vi "stopInPreparePass.vi"(4 "Game in":refnum<class "Game.lvclass">, 7 "OffensivePlay":T1=enum."TestPlay", 8 "error in (no error)":errorcluster, 9 "Ball":refnum<class "Ball.lvclass">, 10 "Robot in":refnum<class "Robot.lvclass">, 11 "AttackerStopTactic in":refnum<class "AttackerStopTactic.lvclass">) -> (0 "error out":errorcluster, 2 "Robot out":refnum<class "Robot.lvclass">, 3 "AttackerStopTactic out":refnum<class "AttackerStopTactic.lvclass">)   [LabVIEW 2023, in "AttackerStopTactic.lvclass"]
uses:
  AttackerStopTactic.lvclass
  Robot_class/Robot.lvclass
  C:/Users/ebert/Desktop/roboime/SSL_AI/Object_class/Object.lvclass
  Ball_class/Ball.lvclass
  Team_class/OffensivePlay.ctl
  Game_class/Game.lvclass
  Utilities_class/Utilities.lvclass
  Game_class/Game.lvclass/Game.ctl
  Object_class/Object.lvclass/Object.ctl
  Robot_class/Robot.lvclass/Robot.ctl
  <vilib>/Analysis/baseanly.llb/Unit Vector (DBL).vi
  Object_class/Read position(x,y).vi
  Object_class/Read y.vi
  Robot_class/Write dest_x.vi
  Robot_class/Write dest_y.vi
  Game_class/Read NewParameters.vi
  <vilib>/Analysis/NI_AALBase.lvlib
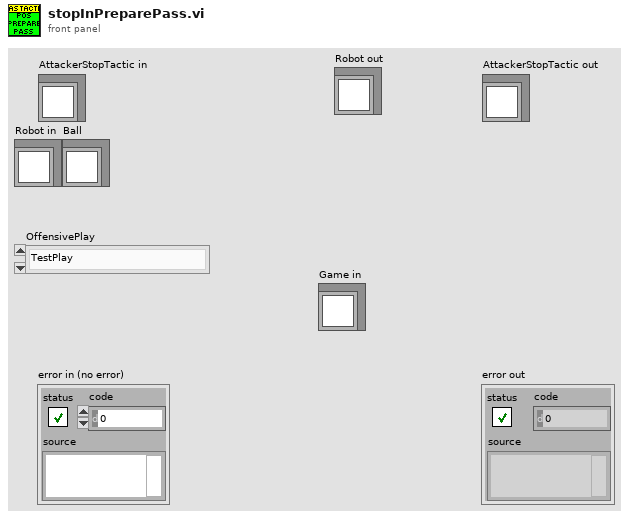
[diagram p1: front panel]
types:
  T1 = typedef "OffensivePlay.ctl" = enum16{"5RobotsPassGamePlay", "5PreparePassGame", "5RobotsKeeperGame", "KeeperPassToStriker", "5RobotsNormalGamePlay", "PrepareKeeperPass", "ACBPass", "ABCPass", "PrepareTriplePass", "TableWithStriker", "TableWith2ndStrikerPlay", "PrepareDoublePass", "PrepareRollToPass", "SimplePass", "PreparePass", "PassToStriker", "BallOutOfField", "PassTo2ndStriker", "StopOffensive", "Prepare Penalty Enemy", "EnemyPossessionAtEnemyField", "EnemyPossesionAtOurField", "TestPlay", "PreparePenaltyAlly", "KickPenaltyAlly", "PrepareKickoffAlly", "PrepareKickoffEnemy", "IndirectEnemy", "DirectEnemy", "PreparePassInGame1", "NormalGame", "DirectKick", "Pass", "Halt", "Timeout", "PassPlay", "PenaltyEnemy"}
  T2 = typedef "NewParameters.ctl" = cluster{"PenaltyDistance":dbl, "DistanceAttackerToBackBall":dbl, "Division":enum16{"Div B", "Div A"}, "DistanceToAvoidyEnemyRobot":dbl, "BallPlacementDistance":dbl, "DisatanceBehindBallToStealBall":dbl, "MaxDistanceToPositionKickoff":dbl, "BlockEnemyTarget":bool, "MaxStopVAng":dbl, "DistanceMarkerToEnemy":dbl, "IgnoreDribblerContact":bool, "DistanceToBeginEnemyPosession":dbl, "GoToBallWhenEnemyNotMoving":bool, "EnemyDistanceToReduceVelocity":dbl, "TurnOnEnemyDistanceToReduceVelocity":bool, "EnemyDistanceToShootOutBall":dbl, "DefenseKickBall":bool, "MoreKickToGoal? (0-0.3)":dbl, "ChipKickInEnemyField":bool, "ShootOutRobotId":dbl, "FieldLenghtDenominatorInShootOut":dbl, "AdjustPositionInBallPlacement":bool, "PowerGodPass":dbl, "VelocityAbortEnemyPos":dbl, "MaxDistToBeginPass":dbl, "MinDistToBeginPass":dbl, "VelocityInDirects":dbl, "BadDribblerIDs":i32[], "NewKickToDistanceAroundBall":dbl, "PowerAvoidColisionMarker":dbl, "DistanceToAvoidColisionMarker":dbl, "AvoidBallKick":dbl, "DistanceTryKick":dbl, "SuicideKickDIstance":dbl, "AdjustFirstKickDistance":dbl, "AvoidAimLessKick":dbl, "DistanceToAvoidyEnemyShootRobot ":dbl, "NumberOfMarkers":dbl, "PotField":bool, "PIDLateral":bool, "MinDistanceFirstKickX":dbl, "MinDistanceFirstKickY":dbl, "FractionOfDistToTouchGround\nAfterChipKick":dbl, "FractionOfKickxWhen\nComposedWithKickz":dbl, "Style":T3, "MoveInTurnState":bool, "DistFromEnemyToConsider\nMoveInTurnState":dbl, "CascadePID":bool, "TurnAroundParameters":cluster{"Radius":dbl, "Multiplier":dbl, "ChordAngle":dbl}, "SafeDriveVel":dbl, "DistanceToGoToBackBall":dbl, "minDistanceToNotFinish\nEnemyPossession":dbl, "OneTouchShot":cluster{"angleFactor":dbl, "maxAngle":dbl, "Attack":bool, "Defense":bool}, "OpenAngleToGoal":cluster{"minAngle":dbl, "maxAngle":dbl, "minEvaluation":dbl}, "ShotInterception":cluster{"shotSpeed":dbl, "minEnemySpeed":dbl, "maxEnemySpeed":dbl, "minEvaluation":dbl}, "AllyTeamArray":T4[], "maxDefendersNumber":i32, "Zone":cluster{"GuardPositionArray":dbl[][], "ZoneMidField":dbl[], "CenterForwardWidth":dbl}, "MinEvaluationToShoot":dbl, "PassInterception":cluster{"maxPassSpeed":dbl, "minPassSpeed":dbl, "minEnemySpeed":dbl, "chipPassDistance":dbl, "chipPassEvaluation":dbl, "minEvaluation":dbl, "maxEnemySpeed":dbl}, "PassDistance":cluster{"maxDistance":dbl, "minDistance":dbl}, "receiverSpeed":dbl, "maxBallSpeed":dbl, "slackTime":dbl, "Turning radius":dbl, "Turning v_ang":dbl, "AlignError":cluster{"Distance":dbl, "Orientation":dbl, "V_norm(m/s)":dbl, "V_ang (rad/s)":dbl}, "RobotRadius":dbl, "KickerDistance":dbl, "keeper angle  to cover goalpost":dbl}
  T3 = typedef "Style.ctl" = enum16{"Insanity", "Offensive", "Defensive"}
  T4 = typedef "AllyTeam.ctl" = enum16{"Keeper", "Defender", "Attacker"}
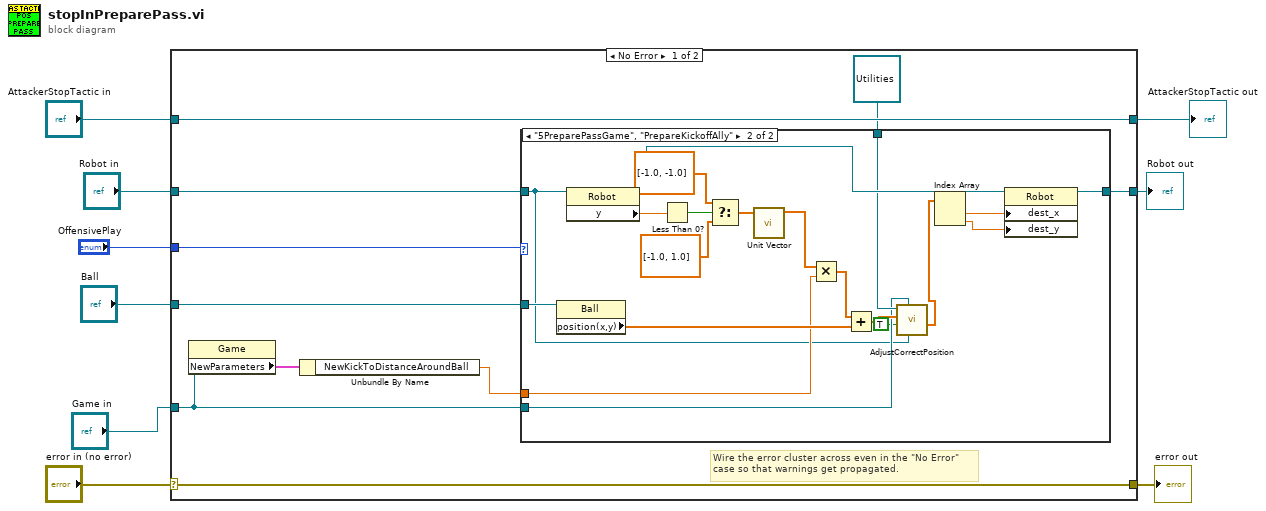
[diagram p0: block diagram]
diagram:
  n1 = case shown="No Error" "error in (no error)" {
    selector: "error in (no error)" -> [w18 w42]
    tunnel: [w18 w42] -> w8
    tunnel: [w19 w41] -> w6
    tunnel: "AttackerStopTactic in" -> [w19 w41]
    tunnel: "Robot in" -> [w17 _]
    tunnel: "Ball" -> [w16 _]
    tunnel: [w15 _] -> w3
    tunnel: "OffensivePlay" -> [w14 _]
    tunnel: "Game in" -> [w12 _]
    frame No Error {
      # "Wire the error cluster across even in the \"No Error\"\ncase so that warnings get propagated."
      n2 = property class="Game"(reference=w12) -> ("NewParameters"=w11:T2)  [unwired: 1 in, 2 out]
      n3 = Unbundle By Name(w11) -> ("NewKickToDistanceAroundBall"=w10:dbl)
      n4 = case shown="\"5PreparePassGame\", \"PrepareKickoffAlly\"" w14 {
        tunnel: w17 -> [w20 w21]
        tunnel: w16 -> [_ w39]
        tunnel: w10 -> [_ w32]
        tunnel: [w20 w27] -> w15
        tunnel: refnum<class "Utilities.lvclass"> refnum ("Utilities in") -> [_ w24]
        tunnel: w12 -> [_ w23]
        frame Default {
        }
        frame "5PreparePassGame", "PrepareKickoffAlly" {
          n5 = property class="Ball"(reference=w39) -> ("position(x,y)"=w38:dbl[])  [unwired: 1 in, 2 out]
          n6 = property class="Robot"(reference=w21) -> (reference out=w30:refnum<class "Robot.lvclass">, "y"=w40:dbl)  [unwired: 1 in, 1 out]
          n7 = Less Than 0?(x=w40) -> (x < 0?=w37:bool)
          n8 = Select(t=dbl[] [-1.0, -1.0], s=w37, f=dbl[] [-1.0, 1.0] ("t")) -> (s? t:f=w34:dbl[])
          n9 = call-poly <vilib>:"Unit Vector.vi"("Input Vector"=w34) -> ("Unit Vector"=w33:dbl[])  [unwired: 8 in, 2 out]
          n10 = Multiply(x=w33, y=w32) -> (x*y=w31:dbl[])
          n11 = Add(x=w31, y=w38) -> (x+y=w26:dbl[])
          n12 = call "AdjustCorrectPosition.vi"("Robot"=w21, "Game"=w23, "IsShoot?"=TRUE, "Position"=w26, "Utilities in"=w24) -> ("AdjustPosition"=w25:dbl[])  [unwired: 4 in, 2 out]
          n13 = Index Array(array=w25) -> (element #1=w29:dbl, element #2=w28:dbl)  [unwired: 2 in]
          n14 = property class="Robot"(reference=w30, "dest_x"=w29, "dest_y"=w28) -> (reference out=w27:refnum<class "Robot.lvclass">)  [unwired: 1 in, 1 out]
        }
      }
    }
    frame Error {
    }
  }
  "error out" <- w8
  "AttackerStopTactic out" <- w6
  "Robot out" <- w3
